vi "anode_timing.vi"(9 "Keep off for X seconds":i32, 10 "Array of timers":dbl[](array[numeric]), 11 "Kill every Y minutes":i32) -> (1 "Time to kill":bool, 2 "Time until reset":dbl, 3 "Time until autokill":dbl, 4 "Time to reset":bool)   [LabVIEW 2018]
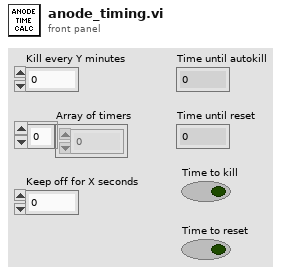
[diagram p1: front panel]
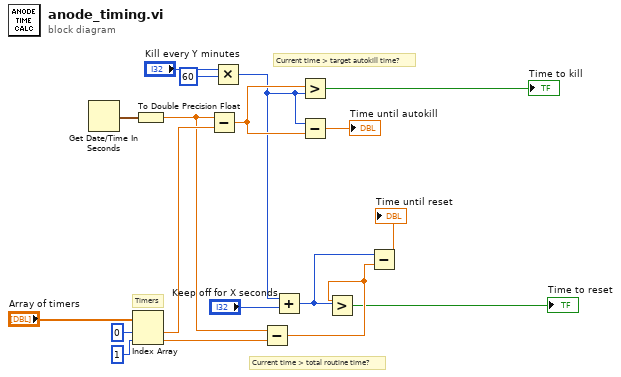
[diagram p0: block diagram]
diagram:
  # "Current time > target autokill time?"
  # "Timers"
  # "Current time > total routine time?"
  n1 = Get Date/Time In Seconds() -> (seconds since 1Jan1904=w2:timestamp)
  n2 = Index Array(array="Array of timers", index #1=0 ("index"), index #2=1 ("index")) -> (element #1=w10:dbl, element #2=w8:dbl)
  n3 = To Double Precision Float(number=w2) -> (double precision float=w9:dbl)
  n4 = Subtract(x=w9, y=w10) -> (x-y=w14:dbl)
  n5 = Multiply(x="Kill every Y minutes", y=60) -> (x*y=w13:i32)
  n6 = Subtract(x=w9, y=w8) -> (x-y=w17:dbl)
  n7 = Add(x=w13, y="Keep off for X seconds") -> (x+y=w16:i32)
  n8 = Greater?(x=w14, y=w13) -> (0:→"Time to kill":bool)
  n9 = Subtract(x=w13, y=w14) -> (x-y=→"Time until autokill":dbl)
  n10 = Greater?(x=w17, y=w16) -> (0:→"Time to reset":bool)
  n11 = Subtract(x=w16, y=w17) -> (x-y=→"Time until reset":dbl)
